vi "Translator.ControlTypeCheck.vi"(1 "control ref":refnum<vi>) -> (0 "control type":T1)   [LabVIEW 2016]
uses:
  Translator.ControlTypes.ctl
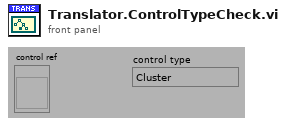
[diagram p1: front panel]
types:
  T1 = typedef "Translator.ControlTypes.ctl" = enum16{"Cluster", "Array", "Boolean", "Ring", "String", "Tab", "Listbox", "Multicolumn listbox", "Table", "Tree", "Other"}
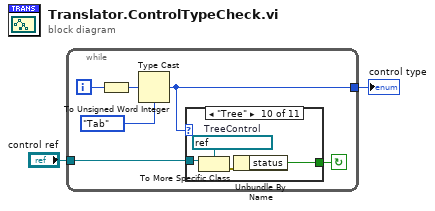
[diagram p0: block diagram]
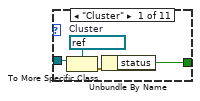
[diagram p2: hidden frame]
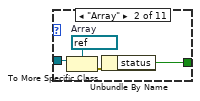
[diagram p3: hidden frame]
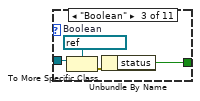
[diagram p4: hidden frame]
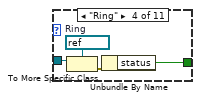
[diagram p5: hidden frame]
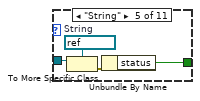
[diagram p6: hidden frame]
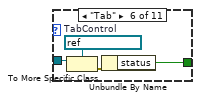
[diagram p7: hidden frame]
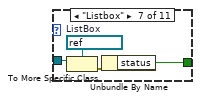
[diagram p8: hidden frame]
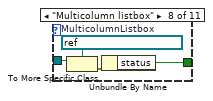
[diagram p9: hidden frame]
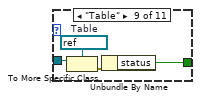
[diagram p10: hidden frame]
diagram:
  n1 = while {
    tunnel: "control ref" -> [w8]
    tunnel: [w5] -> w1
    i -> [w7]
    stop <- w6 continue-if-true
    n2 = To Unsigned Word Integer(number=w7) -> (unsigned 16bit integer=w4:u16)
    n3 = Type Cast(type=Translator.ControlTypes."Tab" ("control type"), x=w4) -> (*(type *) &x=w5:T1)
    n4 = case shown="\"Tree\"" w5 {
      tunnel: w8 -> [w12 w16 w20 w24 w28 w32 w36 w40 w44 w48 _]
      tunnel: [w10 w14 w18 w22 w26 w30 w34 w38 w42 w46 _] -> w6
      frame "Cluster" {
        w9 = refnum<vi> refnum  # Cluster
        n5 = To More Specific Class(target class=w9, reference=w12) -> (error out=w11:errorcluster)  [unwired: 1 in, 1 out]
        n6 = Unbundle By Name(w11) -> ("status"=w10:bool)
      }
      frame "Array" {
        w13 = refnum<vi> refnum  # Array
        n7 = To More Specific Class(target class=w13, reference=w16) -> (error out=w15:errorcluster)  [unwired: 1 in, 1 out]
        n8 = Unbundle By Name(w15) -> ("status"=w14:bool)
      }
      frame "Boolean" {
        w17 = refnum<vi> refnum  # Boolean
        n9 = To More Specific Class(target class=w17, reference=w20) -> (error out=w19:errorcluster)  [unwired: 1 in, 1 out]
        n10 = Unbundle By Name(w19) -> ("status"=w18:bool)
      }
      frame "Ring" {
        w21 = refnum<vi> refnum  # Ring
        n11 = To More Specific Class(target class=w21, reference=w24) -> (error out=w23:errorcluster)  [unwired: 1 in, 1 out]
        n12 = Unbundle By Name(w23) -> ("status"=w22:bool)
      }
      frame "String" {
        w25 = refnum<vi> refnum  # String
        n13 = To More Specific Class(target class=w25, reference=w28) -> (error out=w27:errorcluster)  [unwired: 1 in, 1 out]
        n14 = Unbundle By Name(w27) -> ("status"=w26:bool)
      }
      frame "Tab" {
        w29 = refnum<vi> refnum  # TabControl
        n15 = To More Specific Class(target class=w29, reference=w32) -> (error out=w31:errorcluster)  [unwired: 1 in, 1 out]
        n16 = Unbundle By Name(w31) -> ("status"=w30:bool)
      }
      frame "Listbox" {
        w33 = refnum<vi> refnum  # ListBox
        n17 = To More Specific Class(target class=w33, reference=w36) -> (error out=w35:errorcluster)  [unwired: 1 in, 1 out]
        n18 = Unbundle By Name(w35) -> ("status"=w34:bool)
      }
      frame "Multicolumn listbox" {
        w37 = refnum<vi> refnum  # MulticolumnListbox
        n19 = To More Specific Class(target class=w37, reference=w40) -> (error out=w39:errorcluster)  [unwired: 1 in, 1 out]
        n20 = Unbundle By Name(w39) -> ("status"=w38:bool)
      }
      frame "Table" {
        w41 = refnum<vi> refnum  # Table
        n21 = To More Specific Class(target class=w41, reference=w44) -> (error out=w43:errorcluster)  [unwired: 1 in, 1 out]
        n22 = Unbundle By Name(w43) -> ("status"=w42:bool)
      }
      frame "Tree" {
        w45 = refnum<vi> refnum  # TreeControl
        n23 = To More Specific Class(target class=w45, reference=w48) -> (error out=w47:errorcluster)  [unwired: 1 in, 1 out]
        n24 = Unbundle By Name(w47) -> ("status"=w46:bool)
      }
      frame "Other" {
      }
    }
  }
  "control type" <- w1
